vi "ZMQ.sendMessage.vi"(8 "error in (no error)":errorcluster, 10 "message":T1, 11 "ZMQ":refnum<class "ZMQ_SMO.lvclass">) -> (0 "error out":errorcluster, 3 "ZMQ out":refnum<class "ZMQ_SMO.lvclass">)   [LabVIEW 2016, in "ZMQ_SMO.lvclass"]
doc: "---------------------------------------------------------------\nJKI State Machine Objects™\nhttp://jki.net/state-machine-objects/\nCopyright (C) 2005-2015, JKI <info@jki.net>\nALL RIGHTS RESERVEDJKI State Machine Objects (SMO) 1.0.0.4\nJKI - JKI\nCopyright (c) 2015, JKI"
uses:
  ZMQ_SMO.lvclass
  Typedefs/PrivateEvents--ZMQ.ZMQ_PublicMethod.ctl
  ZMQ_SMO.lvclass/ZMQ_SMO.ctl
panel:
  # "For instructions on how to use the JKI State Machine Objects, examples and video tutorials, visit:\nhttp://jki.net/state-machine-objects/\n\nJKI State Machine Objects™\nhttp://jki.net/state-machine-objects/\nCopyright (C) 2005-2015, JKI <info@jki.net>\nALL RIGHTS RESERVED"
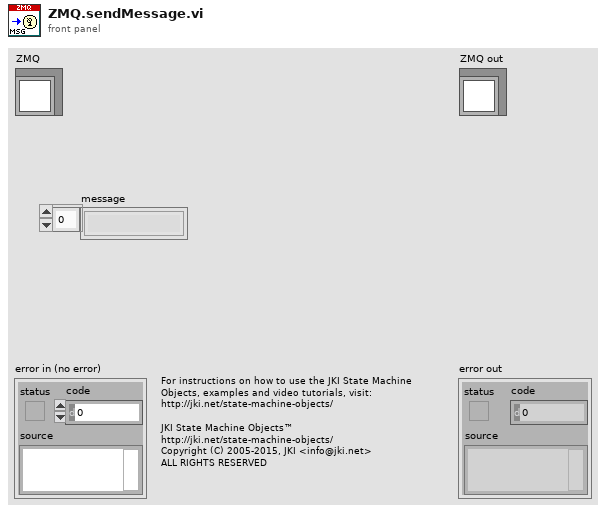
[diagram p1: front panel]
types:
  T1 = typedef "ZMQ_SMO.lvclass/PrivateEvents--ZMQ.ZMQ_PublicMethod.ctl" = string[]
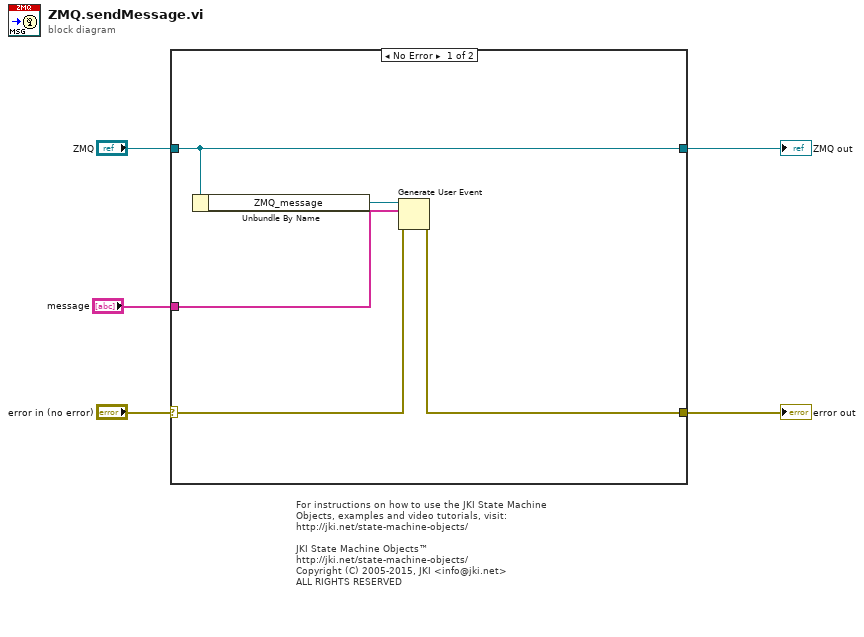
[diagram p0: block diagram]
diagram:
  # "For instructions on how to use the JKI State Machine Objects, examples and video tutorials, visit:\nhttp://jki.net/state-machine-objects/\n\nJKI State Machine Objects™\nhttp://jki.net/state-machine-objects/\nCopyright (C) 2005-2015, JKI <info@jki.net>\nALL RIGHTS RESERVED"
  n1 = case shown="No Error" "error in (no error)" {
    selector: "error in (no error)" -> [w10 w12]
    tunnel: [w7 w12] -> w4
    tunnel: [w6 w11] -> w5
    tunnel: "ZMQ" -> [w6 w11]
    tunnel: "message" -> [w9 _]
    frame No Error {
      n2 = Unbundle By Name(w6) -> ("ZMQ_message"=w8:refnum<user-event>)
      n3 = Generate User Event(user event=w8, event data cluster=w9, error in=w10) -> (error out=w7:errorcluster)  [unwired: 1 in, 1 out]
    }
    frame Error {
    }
  }
  "error out" <- w4
  "ZMQ out" <- w5
